vi "auto_mod.vi"() -> ()   [LabVIEW 2012, in "BlockParty4150.lvrbt"]
uses:
  BlockParty4150.lvrbt
  <vilib>/NXT/Subs/LVHSConnector.ctl
  <vilib>/NXT/LegoClasses/BrickReference/BrickReference.lvclass
  <vilib>/NXT/HiTechnic/HiTechnic Controls/HiTechnic Port.ctl
  <vilib>/NXT/Block Support/NXT_InputPort.ctl
  <vilib>/NXT/Hardware/Plugins/Tetrix 180 deg Servo/Tetrix180ServoAddress.ctl
  <vilib>/NXT/Hardware/Plugins/Tetrix DC Motor/TetrixDCMotorAddress.ctl
  <vilib>/NXT/Dual Mode Library/Display/drawText.vi
  <vilib>/NXT/Dual Mode Library/Sound/Tone.vi
  <vilib>/NXT/NXTIO Xnodes/NXTIONodeSubVIs/TETRIX IO Move DC Motors.vi
  <vilib>/NXT/NXTIO Xnodes/NXTIONodeSubVIs/TETRIX IO Stop DC Motors.vi
  <vilib>/NXT/NXTIO Xnodes/NXTIONodeSubVIs/TETRIX IO Move Servos.vi
  <vilib>/NXT/Dual Mode Library/Waits/Wait_Num(msec).vi
  <vilib>/NXT/NXTIO Xnodes/AddressXNode/NXTIOAddress.xnode
  <vilib>/NXT/NXTIO Xnodes/NXTIOXNode/NXTIO.xnode
panel:
  out "Enabled":bool
  out "iter":i32
  out "NXT":T1
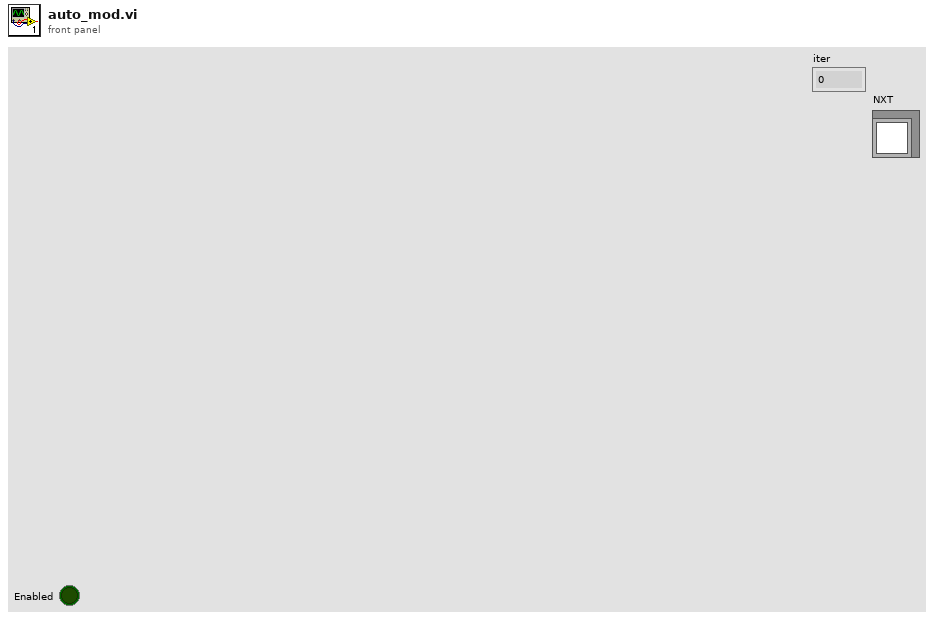
[diagram p1: front panel]
types:
  T1 = typedef "LVHSConnector.ctl" = refnum<class "BrickReference.lvclass">
  T2 = typedef "Tetrix180ServoAddress.ctl" = i16
  T3 = typedef "TetrixDCMotorAddress.ctl" = i16
  T4 = typedef "HiTechnic Port.ctl" = cluster{"Port":T5, "MUX Port":u8}
  T5 = typedef "NXT_InputPort.ctl" = u8
  T6 = cluster{"Direction (0-9)":i16, "Signal Strength (Array)":u8[]}
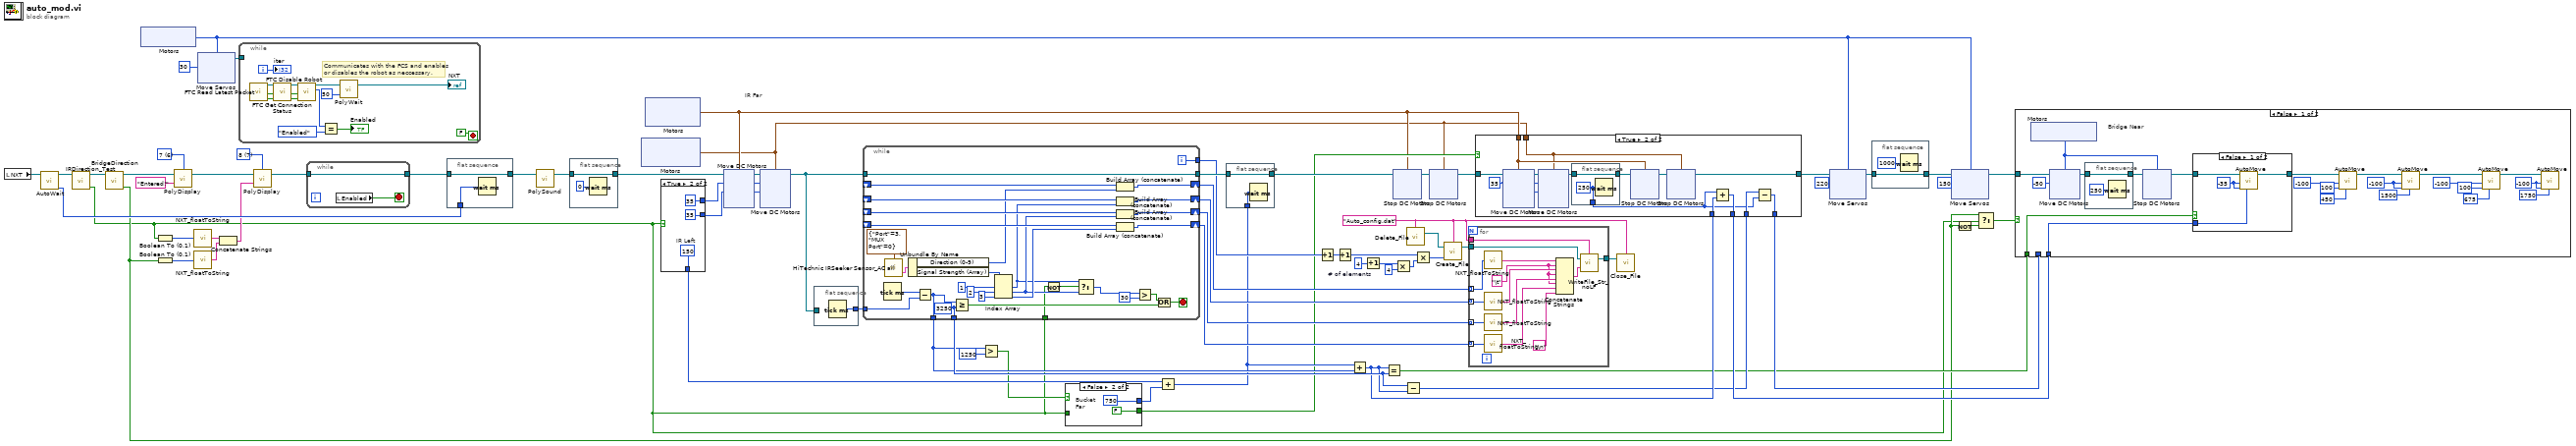
[diagram p0: block diagram]
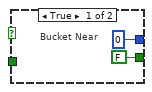
[diagram p3: hidden frame]
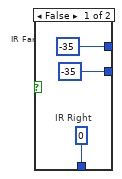
[diagram p4: hidden frame]
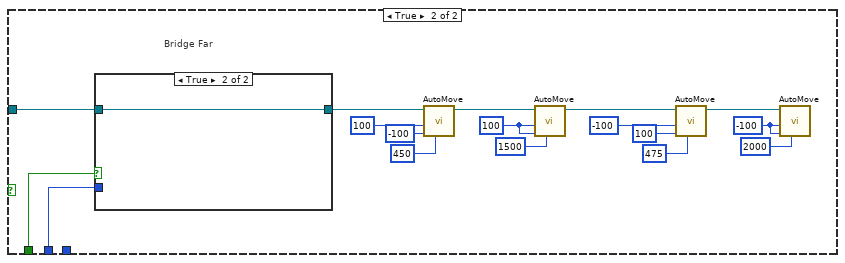
[diagram p6: hidden frame]
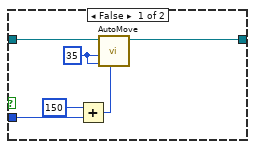
[diagram p7: hidden frame]
diagram:
  w13 = i16 7 items=["1", "2", "3", "4", "5", "6", "7", "8"] ("Line")
  w44 = 4  # # of elements
  w41 = "Auto_config.dat" ("Filename")
  w58 = i16 6 items=["1", "2", "3", "4", "5", "6", "7", "8"] ("Line")
  # "IR Far"
  n1 = local read "NXT"() -> (w69:T1)
  n2 = call "AutoWait.vi"("BrickReference in"=w69) -> ("TimeDelay"=w61:u32, "BrickReference out"=w56:T1)  [unwired: 9 in]
  n3 = call "IRDirection_Test.vi"("BrickReferance In"=w56) -> ("Direction"=w1:bool, "BrickReferance out"=w55:T1)  [unwired: 9 in]
  n4 = call "BridgeDirection.vi"("BrickReference in"=w55) -> ("Direction"=w3:bool, "BrickReference out"=w57:T1)  [unwired: 9 in]
  n5 = xnode "Motors"() -> ("Motor"=w70:T2)
  n6 = Boolean To (0,1)(Boolean=w1) -> (0, 1=w10:i16)
  n7 = Boolean To (0,1)(Boolean=w3) -> (0, 1=w9:i16)
  n8 = call-poly <vilib>:"PolyDisplay.vi"("Text"="Entered!", "NXT"=w57, "Line"=w58) -> ("NXT"=w12:T1)  [unwired: 1 in]
  n9 = call <vilib>:"NXT_floatToString.vi"("number"=w10) -> ("string"=w8:string)
  n10 = call <vilib>:"NXT_floatToString.vi"("number"=w9) -> ("string"=w7:string)
  n11 = xnode "Move Servos"("Position 1"=u8 30, "Servos"=w70) -> ("NXT"=w71:T1)  [unwired: 1 in]
  n12 = Concatenate Strings(w8, w7) -> (w6:string)
  n13 = while {
    tunnel: w71 -> [_]
    i -> [w74]
    stop <- FALSE stop-if-true
    # "Communicates with the FCS and enables \nor disables the robot as neccessary."
    n14 = call <vilib>:"FTC Read Latest Packet.vi"() -> ("Packet Received?"=w84:bool, "Stopped?"=w83:bool, "NXT"=w86:T1)  [unwired: 6 in, 3 out]
    n15 = call <vilib>:"FTC Get Connection Status.vi"("Packet Received?"=w84, "Stopped?"=w83, "NXT"=w86) -> ("Online?"=w76:bool, "Stopped?"=w77:bool, "NXT"=w85:T1)  [unwired: 5 in]
    n16 = call <vilib>:"FTC Disable Robot.vi"("Online?"=w76, "Stopped?"=w77, "NXT"=w85) -> ("Enabled?"=w80:enum16{"Disabled", "Enabled"}, "NXT"=w82:T1)  [unwired: 3 in]
    n17 = Equal?(x=w80, y=enum16{"Disabled", "Enabled"}."Enabled") -> (x = y?=→"Enabled":bool)
    n18 = call-poly <vilib>:"PolyWait.vi"("Time (100 msec)"=u32 50 ("Time (msec)"), "NXT"=w82) -> ("NXT"=→"NXT":T1)  [unwired: 2 in]
    "iter" <- w74
  }
  n19 = call-poly <vilib>:"PolyDisplay.vi"("Text"=w6, "NXT"=w12, "Line"=w13) -> ("NXT"=w11:T1)  [unwired: 1 in]
  n20 = while {
    tunnel: [w88] -> w14
    tunnel: w11 -> [w88]
    stop <- w87 stop-if-true
    n21 = local read "Enabled"() -> (w87:bool)
  }
  n22 = flat-sequence {
    tunnel: w14 -> [w90]
    tunnel: [w90] -> w63
    tunnel: w61 -> [w89]
    frame #0 {
      n23 = Wait (ms)(milliseconds to wait=w89) -> ()  [unwired: 1 out]
    }
  }
  n24 = call-poly <vilib>:"PolySound.vi"("NXT"=w63) -> ("NXT"=w62:T1)  [unwired: 3 in]
  n25 = flat-sequence {
    tunnel: w62 -> [w92]
    tunnel: [w92] -> w68
    frame #0 {
      n26 = Wait (ms)(milliseconds to wait=u32 0) -> ()  [unwired: 1 out]
    }
  }
  n27 = xnode "Motors"() -> ("Motor"=w20:cluster{"TetrixDCMotor":T3, "TetrixDCMotor":T3})
  n28 = xnode "Motors"() -> ("Motor"=w21:cluster{"TetrixDCMotor":T3, "TetrixDCMotor":T3})
  n29 = case shown="True" w1 {
    tunnel: [u32 0 ("milliseconds to wait") u32 150 ("milliseconds to wait")] -> w29
    tunnel: [i8 -35 ("Power/Speed 1") i8 35 ("Power/Speed 1")] -> w54
    tunnel: [i8 -35 ("Power/Speed 1") i8 35 ("Power/Speed 1")] -> w15
    frame False {
      # "IR Right"
      # "IR Far"
    }
    frame True {
      # "IR Left"
    }
  }
  n30 = xnode "Move DC Motors"("Power/Speed 2"=w15, "Power/Speed 1"=w54, "Motors"=w21, "NXT"=w68) -> ("NXT"=w53:T1)
  n31 = xnode "Move DC Motors"("Power/Speed 2"=w15, "Power/Speed 1"=w54, "Motors"=w20, "NXT"=w53) -> ("NXT"=w30:T1)
  n32 = flat-sequence {
    tunnel: [w99] -> w51
    tunnel: w30 -> [_]
    frame #0 {
      n33 = Tick Count (ms)() -> (millisecond timer value=w99:u32)
    }
  }
  n34 = while {
    tunnel: [w129] -> w34
    shift-right: [w128] -> w38
    shift-left: _ -> [w127]
    shift-right: [w125] -> w37
    shift-left: _ -> [w126]
    shift-right: [w115] -> w36
    shift-left: _ -> [w118]
    shift-right: [w114] -> w35
    shift-left: _ -> [w117]
    tunnel: w30 -> [w113]
    tunnel: [w113] -> w50
    tunnel: w51 -> [w109]
    tunnel: [w108] -> w31
    tunnel: [w107] -> w33
    tunnel: w1 -> [w103]
    i -> [w129]
    stop <- w111 stop-if-true
    w107 = u32 3250 ("y")
    n35 = Tick Count (ms)() -> (millisecond timer value=w130:u32)
    n36 = call <vilib>:"HiTechnic IRSeeker Sensor_AC all.vi"("Port/MUX"=T4 {"Port"=3, "MUX Port"=0}) -> ("All Info"=w124:T6)  [unwired: 2 in, 1 out]
    n37 = Unbundle By Name(w124) -> ("Direction (0-9)"=w106:i16, "Signal Strength (Array)"=w123:u8[])
    n38 = Subtract(x=w130, y=w109) -> (x-y=w108:u32)
    n39 = Greater Or Equal?(x=w108, y=w107) -> (x >= y?=w110:bool)
    n40 = Index Array(array=w123, index #1=1 ("index"), index #2=2 ("index"), index #3=3 ("index")) -> (element #1=w102:u8, element #2=w104:u8, element #3=w116:u8)
    n41 = Not(x=w103) -> (.not. x?=w100:bool)
    n42 = Select(t=w102, s=w100, f=w104) -> (s? t:f=w101:u8)
    n43 = Build Array (concatenate)(w127, w106) -> (w128:i16[])
    n44 = Build Array (concatenate)(w126, w102) -> (w125:u8[])
    n45 = Build Array (concatenate)(w118, w104) -> (w115:u8[])
    n46 = Build Array (concatenate)(w117, w116) -> (w114:u8[])
    n47 = Greater?(x=w101, y=u8 30) -> (0:w105:bool)
    n48 = Or(x=w105, y=w110) -> (x .or. y?=w111:bool)
  }
  n49 = Greater?(x=w31, y=u32 1250) -> (0:w25:bool)
  n50 = case shown="False" w25 {
    tunnel: [u32 0 ("y") u32 750 ("y")] -> w26
    tunnel: [FALSE FALSE] -> w24
    tunnel: w1 -> [_ _]
    frame True {
      # "Bucket Near"
    }
    frame False {
      # "Bucket\nFar"
    }
  }
  n51 = Add(x=w29, y=w26) -> (x+y=w27:u32)
  n52 = flat-sequence {
    tunnel: [w136] -> w28
    tunnel: w50 -> [w136]
    tunnel: w27 -> [w135]
    frame #0 {
      n53 = Wait (ms)(milliseconds to wait=w135) -> ()  [unwired: 1 out]
    }
  }
  n54 = Increment(x=w34) -> (x+1=w42:i32)
  n55 = Increment(x=w42) -> (x+1=w48:i32)
  n56 = Add(x=w27, y=w31) -> (x+y=w19:u32)
  n57 = Increment(x=w44) -> (x+1=w45:i32)
  n58 = Equal?(x=w19, y=w33) -> (x = y?=w5:bool)
  n59 = xnode "Stop DC Motors"("Motors"=w21, "NXT"=w28) -> ("NXT"=w52:T1)
  n60 = Multiply(x=w45, y=u32 4) -> (x*y=w46:u32)
  n61 = Subtract(x=w33, y=w19) -> (x-y=w17:u32)
  n62 = call <vilib>:"Delete_File.vi"("Filename"=w41) -> ("NXT"=w49:T1)  [unwired: 3 in]
  n63 = Multiply(x=w48, y=w46) -> (x*y=w39:u32)
  n64 = xnode "Stop DC Motors"("Motors"=w20, "NXT"=w52) -> ("NXT"=w23:T1)
  n65 = call <vilib>:"Create_File.vi"("File Size (256)"=w39, "NXT"=w49, "Filename"=w41) -> ("NXT"=w40:T1)  [unwired: 1 out]
  n66 = for {
    tunnel: w41 -> [w150]
    tunnel: w40 -> [w149]
    tunnel: [w148] -> w43
    tunnel: w38 -> [w147] mode=indexing
    tunnel: w37 -> [w145] mode=indexing
    tunnel: w36 -> [w138] mode=indexing
    tunnel: w35 -> [w137] mode=indexing
    w141 = "\t" ("string")
    n67 = call <vilib>:"NXT_floatToString.vi"("number"=w147) -> ("string"=w144:string)
    n68 = call <vilib>:"NXT_floatToString.vi"("number"=w145) -> ("string"=w143:string)
    n69 = call <vilib>:"NXT_floatToString.vi"("number"=w138) -> ("string"=w142:string)
    n70 = call <vilib>:"NXT_floatToString.vi"("number"=w137) -> ("string"=w140:string)
    n71 = Concatenate Strings(w144, w141, w143, w141, w142, w141, w140, "\n") -> (w146:string)
    n72 = call <vilib>:"WriteFile_Str_noLF.vi"("String"=w146, "NXT"=w149, "Filename"=w150) -> ("NXT"=w148:T1)  [unwired: 1 in]
  }
  n73 = case shown="True" w24 {
    tunnel: [w153 w163] -> w22
    tunnel: w23 -> [w153 w167]
    tunnel: w21 -> [_ w160]
    tunnel: w20 -> [_ w159]
    tunnel: w19 -> [w152 w158]
    tunnel: [w152 w157] -> w18
    tunnel: w17 -> [w151 w156]
    tunnel: [w151 w154] -> w16
    frame False {
    }
    frame True {
      w165 = i8 35 ("Power/Speed 1")
      n74 = xnode "Move DC Motors"("Power/Speed 2"=w165, "Power/Speed 1"=w165, "Motors"=w160, "NXT"=w167) -> ("NXT"=w166:T1)
      n75 = xnode "Move DC Motors"("Power/Speed 2"=w165, "Power/Speed 1"=w165, "Motors"=w159, "NXT"=w166) -> ("NXT"=w164:T1)
      n76 = flat-sequence {
        tunnel: [w183] -> w162
        tunnel: w164 -> [w183]
        tunnel: [w182] -> w155
        frame #0 {
          w182 = u32 250 ("milliseconds to wait")
          n77 = Wait (ms)(milliseconds to wait=w182) -> ()  [unwired: 1 out]
        }
      }
      n78 = xnode "Stop DC Motors"("Motors"=w160, "NXT"=w162) -> ("NXT"=w161:T1)
      n79 = xnode "Stop DC Motors"("Motors"=w159, "NXT"=w161) -> ("NXT"=w163:T1)
      n80 = Add(x=w155, y=w158) -> (x+y=w157:u32)
      n81 = Subtract(x=w156, y=w155) -> (x-y=w154:u32)
      n82 = flat-sequence {
        frame #0 {
          n83 = Wait (ms)(milliseconds to wait=u32 1000) -> ()  [unwired: 1 out]
        }
      }
    }
  }
  n84 = call <vilib>:"Close_File.vi"("NXT"=w43, "Filename"=w41) -> ()  [unwired: 2 in, 1 out]
  n85 = xnode "Move Servos"("Position 1"=u8 220, "Servos"=w70, "NXT"=w22) -> ("NXT"=w66:T1)
  n86 = flat-sequence {
    tunnel: [w205] -> w64
    tunnel: w66 -> [w205]
    frame #0 {
      n87 = Wait (ms)(milliseconds to wait=u32 1000) -> ()  [unwired: 1 out]
    }
  }
  n88 = xnode "Move Servos"("Position 1"=u8 150, "Servos"=w70, "NXT"=w64) -> ("NXT"=w60:T1)
  n89 = Not(x=w3) -> (.not. x?=w2:bool)
  n90 = Select(t=w3, s=w1, f=w2) -> (s? t:f=w4:bool)
  n91 = case shown="False" w4 {
    tunnel: w16 -> [_ w249]
    tunnel: w5 -> [w214 w252]
    tunnel: w60 -> [w208 w250]
    tunnel: w18 -> [w207 _]
    frame False {
      w223 = i8 -100 ("Left Power")
      w218 = i8 -100 ("Left Power")
      # "Bridge Near"
      n92 = xnode "Motors"() -> ("Motor"=w209:T3)
      n93 = xnode "Move DC Motors"("Power/Speed 1"=i8 -50, "Motors"=w209, "NXT"=w208) -> ("NXT"=w212:T1)
      n94 = flat-sequence {
        tunnel: [w234] -> w211
        tunnel: w212 -> [w234]
        frame #0 {
          n95 = Wait (ms)(milliseconds to wait=u32 250) -> ()  [unwired: 1 out]
        }
      }
      n96 = xnode "Stop DC Motors"("Motors"=w209, "NXT"=w211) -> ("NXT"=w210:T1)
      n97 = case shown="False" w214 {
        tunnel: w207 -> [w244 _]
        tunnel: [w245 w248] -> w228
        tunnel: w210 -> [w246 w248]
        frame False {
          w247 = i8 -35 ("Left Power")
          n98 = call "AutoMove.vi"("Wait"=w244, "Right Power"=w247, "Left Power"=w247, "BrickReference in"=w246) -> ("BrickReference out"=w245:T1)  [unwired: 7 in]
        }
        frame True {
        }
      }
      n99 = call "AutoMove.vi"("Wait"=u32 450, "Right Power"=i8 100, "Left Power"=i8 -100, "BrickReference in"=w228) -> ("BrickReference out"=w227:T1)  [unwired: 7 in]
      n100 = call "AutoMove.vi"("Wait"=u32 1500, "Right Power"=w218, "Left Power"=w218, "BrickReference in"=w227) -> ("BrickReference out"=w225:T1)  [unwired: 7 in]
      n101 = call "AutoMove.vi"("Wait"=u32 675, "Right Power"=i8 100, "Left Power"=i8 -100, "BrickReference in"=w225) -> ("BrickReference out"=w226:T1)  [unwired: 7 in]
      n102 = call "AutoMove.vi"("Wait"=u32 1750, "Right Power"=w223, "Left Power"=w223, "BrickReference in"=w226) -> ()  [unwired: 7 in, 1 out]
    }
    frame True {
      w257 = i8 -100 ("Left Power")
      w262 = i8 100 ("Left Power")
      # "Bridge Far"
      n103 = case shown="True" w252 {
        tunnel: w249 -> [w269 _]
        tunnel: [w267 w272] -> w251
        tunnel: w250 -> [w268 w272]
        frame False {
          w271 = i8 35 ("Left Power")
          n104 = Add(x=u32 150, y=w269) -> (x+y=w270:u32)
          n105 = call "AutoMove.vi"("Wait"=w270, "Right Power"=w271, "Left Power"=w271, "BrickReference in"=w268) -> ("BrickReference out"=w267:T1)  [unwired: 7 in]
        }
        frame True {
        }
      }
      n106 = call "AutoMove.vi"("Wait"=u32 450, "Right Power"=i8 -100, "Left Power"=i8 100, "BrickReference in"=w251) -> ("BrickReference out"=w253:T1)  [unwired: 7 in]
      n107 = call "AutoMove.vi"("Wait"=u32 1500, "Right Power"=w262, "Left Power"=w262, "BrickReference in"=w253) -> ("BrickReference out"=w255:T1)  [unwired: 7 in]
      n108 = call "AutoMove.vi"("Wait"=u32 475, "Right Power"=i8 100, "Left Power"=i8 -100, "BrickReference in"=w255) -> ("BrickReference out"=w254:T1)  [unwired: 7 in]
      n109 = call "AutoMove.vi"("Wait"=u32 2000, "Right Power"=w257, "Left Power"=w257, "BrickReference in"=w254) -> ()  [unwired: 7 in, 1 out]
    }
  }
